vi "Set Cell Value (Boolean).vi"(8 "error in":errorcluster, 9 "Value":bool, 10 "Cell Address":string, 11 "WorksheetPart in":refnum<k24>) -> (0 "error out":errorcluster, 3 "WorksheetPart out":refnum<k24>)   [LabVIEW 2019, in "Open Xml.lvlib"]
uses:
  Open Xml.lvlib
  D:/git/Open-Xml-LabVIEW/Source/DocumentFormat.OpenXml.dll
  DocumentFormat.OpenXml.dll
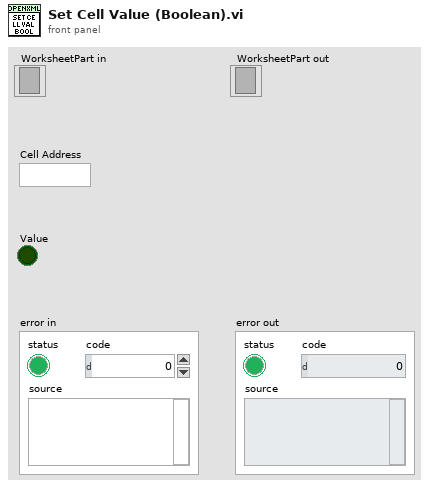
[diagram p1: front panel]
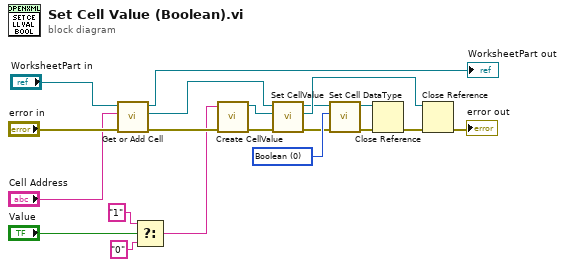
[diagram p0: block diagram]
diagram:
  w7 = 0 items=["Boolean", "Number", "Error", "SharedString", "String", "InlineString", "Date"] ("Datatype")
  n1 = call "Get or Add Cell.vi"("error in"="error in", "Cell Address"="Cell Address", "Worksheetpart in"="WorksheetPart in") -> ("error out"=w15:errorcluster, "Cell"=w9:refnum<k24>, "WorksheetPart out"=→"WorksheetPart out":refnum<k24>)  [unwired: 6 in]
  n2 = Select(t="1", s="Value", f="0" ("t")) -> (s? t:f=w12:string)
  n3 = call "Create CellValue.vi"("error in"=w15, "Text"=w12) -> ("error out"=w3:errorcluster, "CellValue out"=w8:refnum<k24>)  [unwired: 8 in]
  n4 = call "Set CellValue.vi"("error in"=w3, "CellValue in"=w8, "Cell in"=w9) -> ("error out"=w6:errorcluster, "CellValue out"=w20:refnum<k24>, "Cell out"=w5:refnum<k24>)  [unwired: 6 in]
  n5 = call "Set Cell DataType.vi"("error in"=w6, "Datatype"=w7, "Cell in"=w5) -> ("error out"=w4:errorcluster, "Cell out"=w19:refnum<k24>)  [unwired: 7 in]
  n6 = Close Reference(reference=w19, error in (no error)=w4) -> (error out=w18:errorcluster)
  n7 = Close Reference(reference=w20, error in (no error)=w18) -> (error out=→"error out":errorcluster)
